vi "Move and Hide String Item.vi"(8 "error in (no error)":errorcluster, 11 "String in":refnum<vi>) -> (0 "error out":errorcluster)   [LabVIEW 2013, in "CANopen Workspace Objects.lvlib"]
uses:
  CANopen Workspace Objects.lvlib
  <vilib>/Utility/miscctls.llb/LVPositionTypeDef.ctl
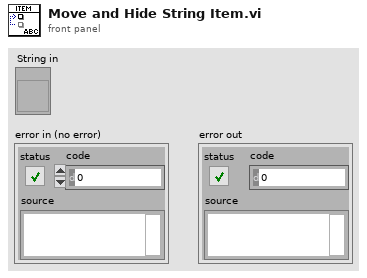
[diagram p1: front panel]
types:
  T1 = typedef "LVPositionTypeDef.ctl" = cluster{"Left":i32, "Top":i32}
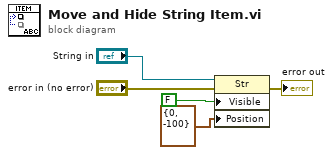
[diagram p0: block diagram]
diagram:
  n1 = property class="Str"(reference="String in", error in="error in (no error)", "Visible"=FALSE, "Position"=T1 {"Left"=0, "Top"=-100}) -> (error out=→"error out":errorcluster)  [unwired: 1 out]
